vi "Auto Execute Commands.vi"(11 "Auto Command":T1[](array[typedef])) -> ()   [LabVIEW 2019]
uses:
  Controls/Auto Controls.ctl
  <vilib>/Rock Robotics/WPI/Solenoid/WPI_SolenoidValue.ctl
  <vilib>/Rock Robotics/WPI/Solenoid/WPI_SolenoidSetEnum.vi
  Framework/Robot Global Data.vi
panel:
  out "File Recorded":T2(ring)
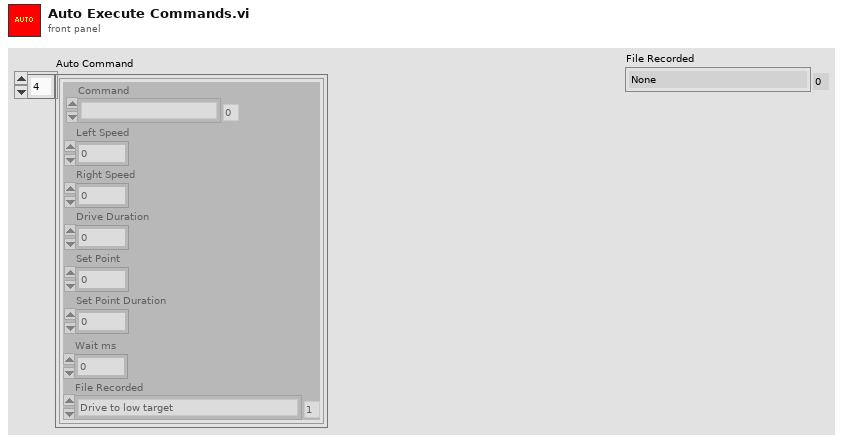
[diagram p1: front panel]
types:
  T1 = typedef "Auto Controls.ctl" = cluster{"Drive Duration":dbl, "Left Speed":dbl, "Right Speed":dbl, "Set Point":dbl, "Set Point Duration":dbl, "Command":enum16{"", "Drive Forwards", "Drive Backwards", "Stop", "Turn Left", "Turn Right", "Drop Intake", "Lift Intake", "Intake", "Shooter", "Transfer", "Wait", "Drive from recorded file"}, "Wait ms":dbl, "File Recorded":enum16{"None", "Drive to low target", "Drive to pick balls from the right CP", "Drive to pick up balls from the Left CP", "Drive to pick up 3 balls from the center", "Drive to pick up 2 balls from the center"}}
  T2 = enum16{"None", "Drive to low target", "Drive to pick balls from the right CP", "Drive to pick up balls from the Left CP", "Drive to pick up 3 balls from the center", "Drive to pick up 2 balls from the center"}
  T3 = typedef "WPI_SolenoidValue.ctl" = enum16{"Off", "On", "Forward", "Reverse"}
  T4 = enum16{"", "Drive Forwards", "Drive Backwards", "Stop", "Turn Left", "Turn Right", "Drop Intake", "Lift Intake", "Intake", "Shooter", "Transfer", "Wait", "Drive from recorded file"}
  T5 = typedef "WPI_SolenoidDevRef.ctl" = cluster{"DevStatus":errorcluster, "Pneumatics Control Module":u8, "Forward Solenoid Channel":T6, "Reverse Solenoid Channel":T6}
  T6 = typedef "WPI_SolenoidChannel.ctl" = enum8{"Solenoid 0", "Solenoid 1", "Solenoid 2", "Solenoid 3", "Solenoid 4", "Solenoid 5", "Solenoid 6", "Solenoid 7", "Invalid"}
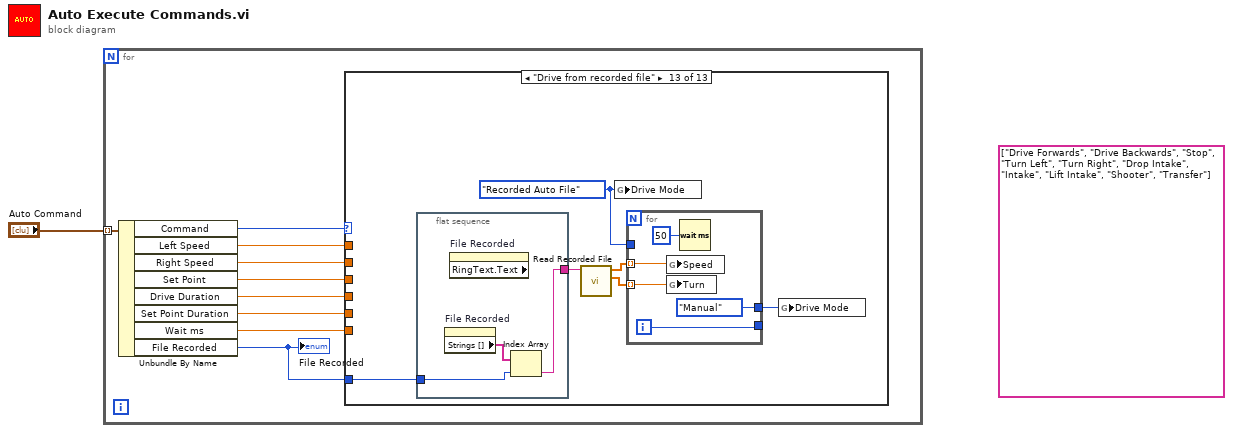
[diagram p0: block diagram]
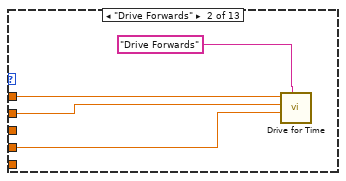
[diagram p3: hidden frame]
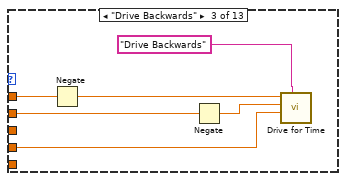
[diagram p4: hidden frame]
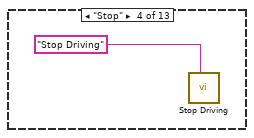
[diagram p5: hidden frame]
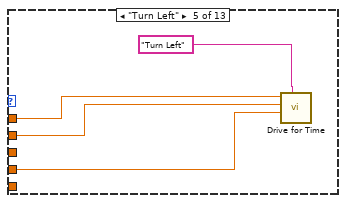
[diagram p6: hidden frame]
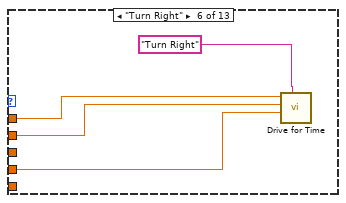
[diagram p7: hidden frame]
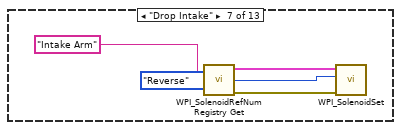
[diagram p8: hidden frame]
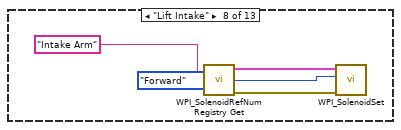
[diagram p9: hidden frame]
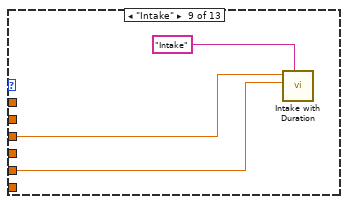
[diagram p10: hidden frame]
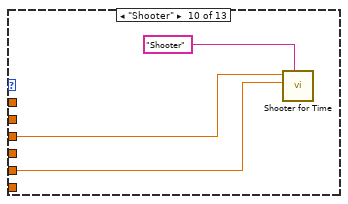
[diagram p11: hidden frame]
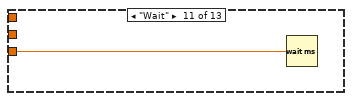
[diagram p12: hidden frame]
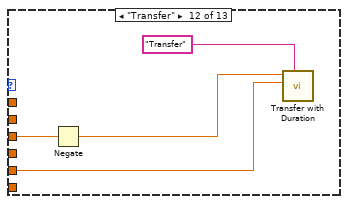
[diagram p13: hidden frame]
diagram:
  (unwired) string[] ["Drive Forwards", "Drive Backwards", "Stop", "Turn Left", "Turn Right", "Drop Intake", "Intake", "Lift Intake", "Shooter", "Transfer"]
  n1 = for {
    tunnel: "Auto Command" -> [w10] mode=indexing
    n2 = Unbundle By Name(w10) -> ("Command"=w9:T4, "Left Speed"=w8:dbl, "Right Speed"=w7:dbl, "Set Point"=w5:dbl, "Drive Duration"=w6:dbl, "Set Point Duration"=w4:dbl, "Wait ms"=w3:dbl, "File Recorded"=w2:T2)
    "File Recorded" <- w2
    n3 = case shown="\"Drive from recorded file\"" w9 {
      tunnel: w8 -> [_ w13 w19 _ w24 w28 _ _ _ _ _ _ _]
      tunnel: w7 -> [_ w12 w18 _ w23 w27 _ _ _ _ _ _ _]
      tunnel: w6 -> [_ w11 w17 _ w22 w26 _ _ _ _ _ _ _]
      tunnel: w5 -> [_ _ _ _ _ _ _ _ w39 w42 _ w47 _]
      tunnel: w4 -> [_ _ _ _ _ _ _ _ w38 w41 _ w45 _]
      tunnel: w3 -> [_ _ _ _ _ _ _ _ _ _ w44 _ _]
      tunnel: w2 -> [_ _ _ _ _ _ _ _ _ _ _ _ w49]
      frame Default {
      }
      frame "Drive Forwards" {
        n4 = call "Drive for Time.vi"("Description"="Drive Forwards", "Seconds"=w11, "Right Speed"=w12, "Left Speed"=w13) -> ()  [unwired: 7 in, 1 out]
      }
      frame "Drive Backwards" {
        n5 = Negate(x=w19) -> (-x=w16:dbl)
        n6 = Negate(x=w18) -> (-x=w15:dbl)
        n7 = call "Drive for Time.vi"("Description"="Drive Backwards", "Seconds"=w17, "Right Speed"=w15, "Left Speed"=w16) -> ()  [unwired: 7 in, 1 out]
      }
      frame "Stop" {
        n8 = call "Stop Driving.vi"("Description"="Stop Driving") -> ()  [unwired: 10 in, 1 out]
      }
      frame "Turn Left" {
        n9 = call "Drive for Time.vi"("Description"="Turn Left", "Seconds"=w22, "Right Speed"=w23, "Left Speed"=w24) -> ()  [unwired: 7 in, 1 out]
      }
      frame "Turn Right" {
        n10 = call "Drive for Time.vi"("Description"="Turn Right", "Seconds"=w26, "Right Speed"=w27, "Left Speed"=w28) -> ()  [unwired: 7 in, 1 out]
      }
      frame "Drop Intake" {
        n11 = call <vilib>:"WPI_SolenoidRefNum Registry Get.vi"("refnum name"="Intake Arm") -> ("error out"=w31:errorcluster, "SolenoidDevRef"=w32:T5)  [unwired: 9 in]
        n12 = call-poly <vilib>:"WPI_SolenoidSet.vi"("error in (no error)"=w31, "Value"=WPI_SolenoidValue."Reverse", "SolenoidDevRef"=w32) -> ()  [unwired: 7 in, 2 out]
      }
      frame "Lift Intake" {
        n13 = call <vilib>:"WPI_SolenoidRefNum Registry Get.vi"("refnum name"="Intake Arm") -> ("error out"=w35:errorcluster, "SolenoidDevRef"=w36:T5)  [unwired: 9 in]
        n14 = call-poly <vilib>:"WPI_SolenoidSet.vi"("error in (no error)"=w35, "Value"=WPI_SolenoidValue."Forward", "SolenoidDevRef"=w36) -> ()  [unwired: 7 in, 2 out]
      }
      frame "Intake" {
        n15 = call "Intake with Duration.vi"("Description"="Intake", "Duration (s)"=w38, "Setpoint"=w39) -> ()  [unwired: 8 in, 1 out]
      }
      frame "Shooter" {
        n16 = call "Shooter for Time.vi"("Description"="Shooter", "Duration (s)"=w41, "Setpoint"=w42) -> ()  [unwired: 8 in, 1 out]
      }
      frame "Wait" {
        n17 = Wait (ms)(milliseconds to wait=w44) -> ()  [unwired: 1 out]
      }
      frame "Transfer" {
        n18 = Negate(x=w47) -> (-x=w46:dbl)
        n19 = call "Transfer with Duration.vi"("Description"="Transfer", "Duration (s)"=w45, "Setpoint"=w46) -> ()  [unwired: 8 in, 1 out]
      }
      frame "Drive from recorded file" {
        w54 = enum16{"Manual", "Recorded Auto File"}."Recorded Auto File" ("Drive Mode")
        n20 = flat-sequence {
          tunnel: [w55] -> w50
          tunnel: w49 -> [w56]
          frame #0 {
            n21 = property on="File Recorded" class="Enum (strict)"() -> ("Strings []"=w57:string[])  [unwired: 2 in, 2 out]
            n22 = property on="File Recorded" class="Enum (strict)" props=["RingText", "Text"]() -> ()  [unwired: 2 in, 3 out]
            n23 = Index Array(array=w57, index=w56) -> (element=w55:string)
          }
        }
        n24 = call "Read Recorded File.vi"("Filename"=w50) -> ("Turn"=w52:dbl[], "Speed"=w51:dbl[])  [unwired: 9 in]
        n25 = global write "Robot Global Data.vi" "Drive Mode"(w54) -> ()
        n26 = for {
          tunnel: w51 -> [w62] mode=indexing
          tunnel: w52 -> [w61] mode=indexing
          tunnel: [enum16{"Manual", "Recorded Auto File"}."Manual" ("Drive Mode")] -> w53
          tunnel: w54 -> [_]
          tunnel: [w58] -> _
          i -> [w58]
          n27 = global write "Robot Global Data.vi" "Speed"(w62) -> ()
          n28 = global write "Robot Global Data.vi" "Turn"(w61) -> ()
          n29 = Wait (ms)(milliseconds to wait=u32 50) -> ()  [unwired: 1 out]
        }
        n30 = global write "Robot Global Data.vi" "Drive Mode"(w53) -> ()
      }
    }
  }
